vi "Update graph.vi"(6 "X and Y scaling":dbl[](array[numeric]), 7 "Set Axis Scale?":bool, 8 "error in (no error)":errorcluster, 9 "Template?":bool=TRUE, 10 "Data":cluster{"X Data":dbl[], "Y Data":dbl[]}, 11 "Data Viewer in":refnum<class "Lissajous Viewer.lvclass">) -> (0 "error out":errorcluster, 3 "Data Viewer out":refnum<class "Lissajous Viewer.lvclass">)   [LabVIEW 2020, in "Lissajous Viewer.lvlib" / "Lissajous Viewer.lvclass"]
doc: "Initializes the Data Viewer Panel Actor.\n----\nCopyright: MGI 2017\nAuthor: Derek Trepanier"
uses:
  Lissajous Viewer.lvclass
  Lissajous Viewer.lvclass/Lissajous Viewer.ctl
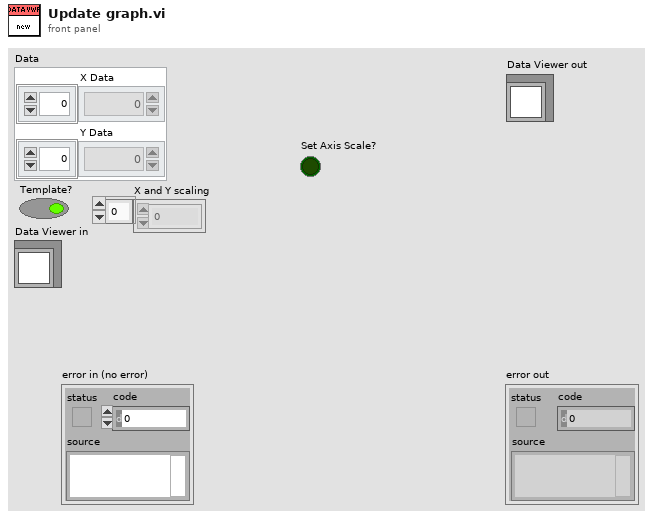
[diagram p1: front panel]
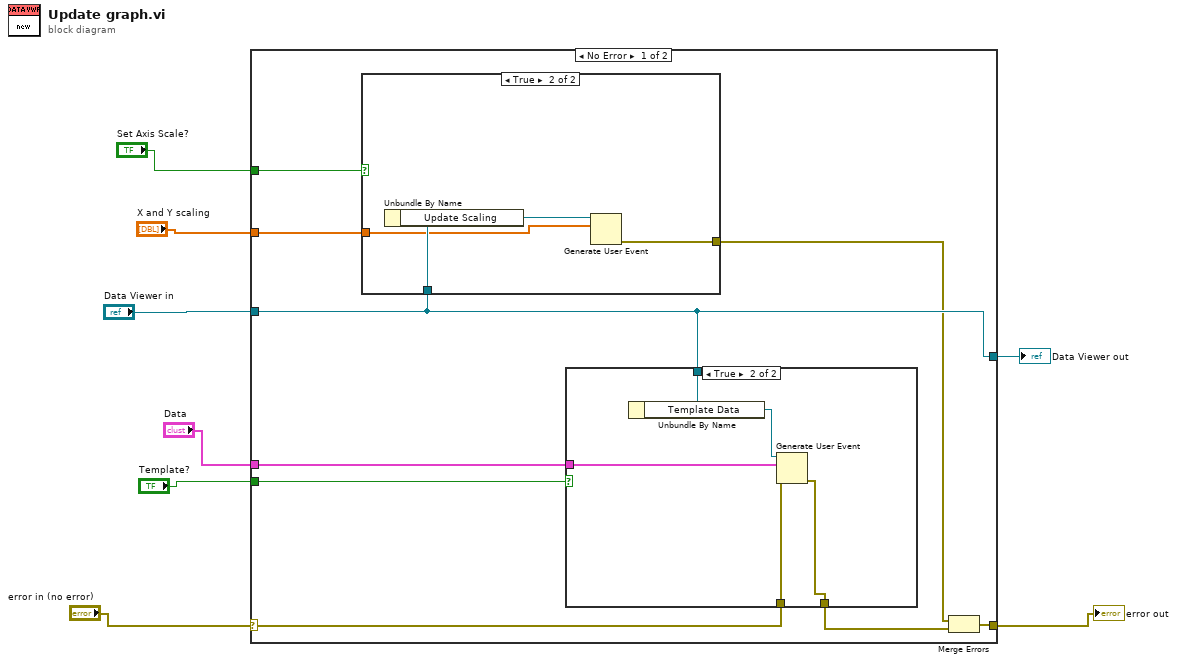
[diagram p0: block diagram]
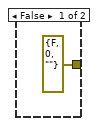
[diagram p2: hidden frame]
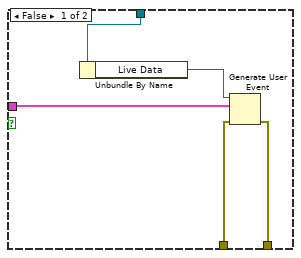
[diagram p3: hidden frame]
diagram:
  n1 = case shown="No Error" "error in (no error)" {
    selector: "error in (no error)" -> [w15 w34]
    tunnel: "Data Viewer in" -> [w13 w33]
    tunnel: [w13 w33] -> w7
    tunnel: [w12 w34] -> w5
    tunnel: "Template?" -> [w17 _]
    tunnel: "Data" -> [w16 _]
    tunnel: "Set Axis Scale?" -> [w14 _]
    tunnel: "X and Y scaling" -> [w9 _]
    frame No Error {
      n2 = case shown="True" w14 {
        tunnel: w13 -> [_ w22]
        tunnel: [errorcluster {"status"=FALSE, "code"=0, "source"=""} ("error out") w20] -> w10
        tunnel: w9 -> [_ w19]
        frame False {
        }
        frame True {
          n3 = Unbundle By Name(w22) -> ("Update Scaling"=w21:refnum<user-event>)
          n4 = Generate User Event(user event=w21, event data cluster=w19) -> (error out=w20:errorcluster)  [unwired: 2 in, 1 out]
        }
      }
      n5 = case shown="True" w17 {
        tunnel: w13 -> [w27 w32]
        tunnel: w16 -> [w25 w30]
        tunnel: w15 -> [w24 w29]
        tunnel: [w23 w28] -> w11
        frame False {
          n6 = Unbundle By Name(w27) -> ("Live Data"=w26:refnum<user-event>)
          n7 = Generate User Event(user event=w26, event data cluster=w25, error in=w24) -> (error out=w23:errorcluster)  [unwired: 1 in, 1 out]
        }
        frame True {
          n8 = Unbundle By Name(w32) -> ("Template Data"=w31:refnum<user-event>)
          n9 = Generate User Event(user event=w31, event data cluster=w30, error in=w29) -> (error out=w28:errorcluster)  [unwired: 1 in, 1 out]
        }
      }
      n10 = Merge Errors(w10, w11) -> (w12:errorcluster)
    }
    frame Error {
    }
  }
  "error out" <- w5
  "Data Viewer out" <- w7
